vi "Build New Member Path.vi"(10 "Member Name":string, 11 "Class":refnum<vi>) -> (2 "New Member Name":string, 3 "New Member Path":path)   [LabVIEW 2018, in "LVClassByRef.lvlib"]
uses:
  <resource>/Framework/Providers/LVClassByRef/LVClassByRef.lvlib
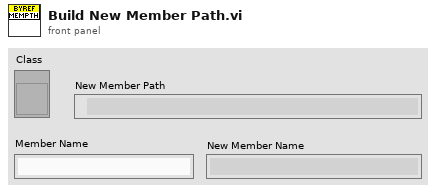
[diagram p1: front panel]
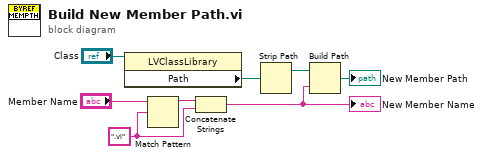
[diagram p0: block diagram]
diagram:
  w2 = ".vi" ("regular expression")
  n1 = property class="LVClassLibrary"(reference="Class") -> ("Path"=w7:path)  [unwired: 1 in, 2 out]
  n2 = Match Pattern(string="Member Name", regular expression=w2) -> (before substring=w3:string)  [unwired: 1 in, 3 out]
  n3 = Concatenate Strings(w3, w2) -> (w1:string)
  "New Member Name" <- w1
  n4 = Strip Path(path=w7) -> (stripped path=w6:path)  [unwired: 1 out]
  n5 = Build Path(base path=w6, name or relative path=w1) -> (appended path=→"New Member Path":path)
